vi "图像交错组合与分离.vi"() -> ()   [LabVIEW 2018]
uses:
  <vilib>/vision/NI_Vision_Development_Module.lvlib
panel:
  out "error out":errorcluster
  out "Image":T1(plugin-control)
  in  "路径":path
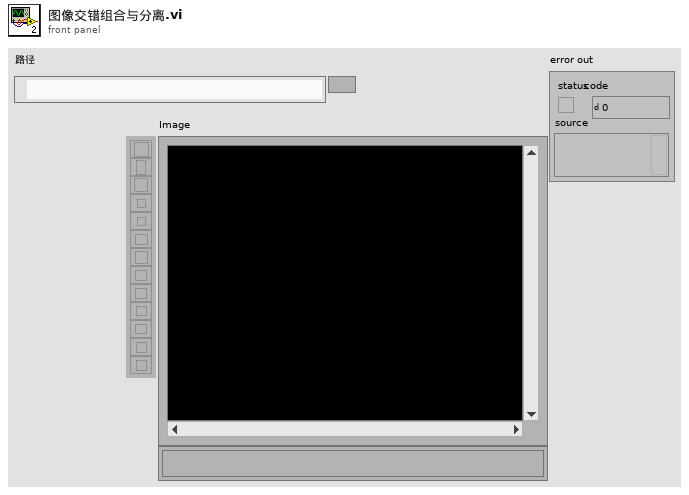
[diagram p1: front panel]
types:
  T1 = typedef "IMAQ Image.ctl" = refnum<image>
  T2 = typedef "Image Type" = u32
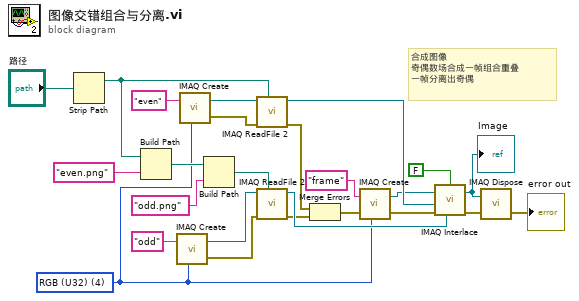
[diagram p0: block diagram]
diagram:
  w1 = T2 4 items=["Grayscale (U8)", "Grayscale (I16)", "Grayscale (SGL)", "Complex (CSG)", "RGB (U32)", "HSL (U32)", "RGB (U64)", "Grayscale (U16)"] ("Image Type")
  # "合成图像\n奇偶数场合成一帧组合重叠\n一帧分离出奇偶"
  n1 = Strip Path(path="路径") -> (stripped path=w15:path)  [unwired: 1 out]
  n2 = Build Path(base path=w15, name or relative path="even.png" ("名称或相对路径")) -> (appended path=w23:path)
  n3 = call "IMAQ Create"("Image Name"="odd", "Image Type"=w1) -> ("New Image"=w19:T1, "error out"=w18:errorcluster)  [unwired: 3 in]
  n4 = call "IMAQ Create"("Image Name"="even", "Image Type"=w1) -> ("New Image"=w16:T1, "error out"=w17:errorcluster)  [unwired: 3 in]
  n5 = Build Path(base path=w23, name or relative path="odd.png" ("名称或相对路径")) -> (appended path=w14:path)
  n6 = call "IMAQ ReadFile 2"("File Path"=w15, "error in (no error)"=w17, "Image"=w16) -> ("error out"=w7:errorcluster, "Image Out"=w13:T1)  [unwired: 4 in, 3 out]
  n7 = call "IMAQ ReadFile 2"("File Path"=w14, "error in (no error)"=w18, "Image"=w19) -> ("error out"=w6:errorcluster, "Image Out"=w12:T1)  [unwired: 4 in, 3 out]
  n8 = Merge Errors(w7, w6) -> (w8:errorcluster)
  n9 = call "IMAQ Create"("Image Name"="frame", "Image Type"=w1, "error in (no error)"=w8) -> ("New Image"=w10:T1, "error out"=w5:errorcluster)  [unwired: 2 in]
  n10 = call "IMAQ Interlace"("error in (no error)"=w5, "Image Even"=w13, "Image Odd"=w12, "Image Frame"=w10, "Interlace/Separate (Interlace)"=FALSE) -> ("error out"=w4:errorcluster, "Image Frame Out"=w3:T1)  [unwired: 2 out]
  "Image" <- w3
  n11 = call "IMAQ Dispose"("Image"=w3, "error in (no error)"=w4) -> ("error out"=→"error out":errorcluster)  [unwired: 4 in]
